vi "WPI_DMAEnableGlobal.vi"(9 "Set":bool, 10 "DMA Enable":T1) -> (1 "WordsPerSample":u16, 2 "DMA Enable Out":T1)   [LabVIEW 2017]
uses:
  <vilib>/Rock Robotics/SystemInterfaces/DMA/FPGA_DMAEnable.ctl
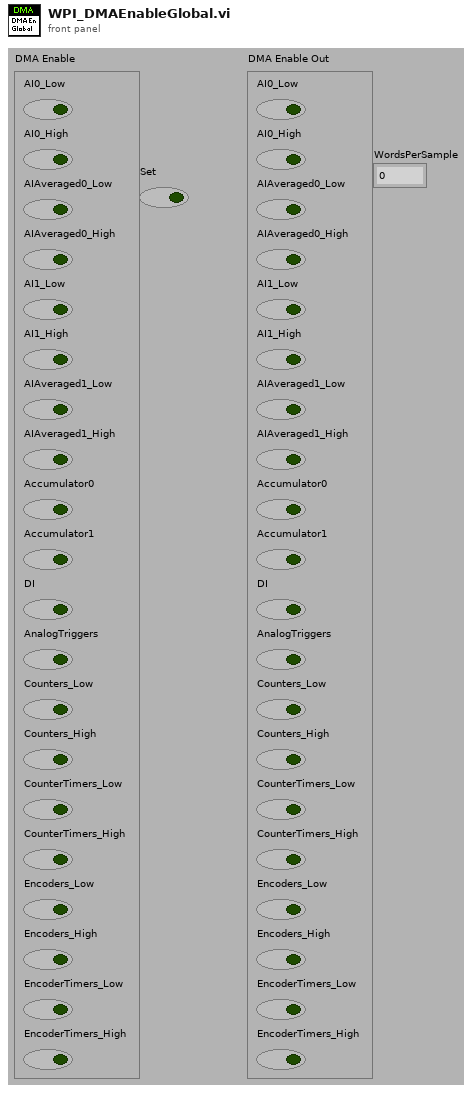
[diagram p1: front panel]
types:
  T1 = typedef "FPGA_DMAEnable.ctl" = cluster{"AI0_Low":bool, "AI0_High":bool, "AIAveraged0_Low":bool, "AIAveraged0_High":bool, "AI1_Low":bool, "AI1_High":bool, "AIAveraged1_Low":bool, "AIAveraged1_High":bool, "Accumulator0":bool, "Accumulator1":bool, "DI":bool, "AnalogTriggers":bool, "Counters_Low":bool, "Counters_High":bool, "CounterTimers_Low":bool, "CounterTimers_High":bool, "Encoders_Low":bool, "Encoders_High":bool, "EncoderTimers_Low":bool, "EncoderTimers_High":bool}
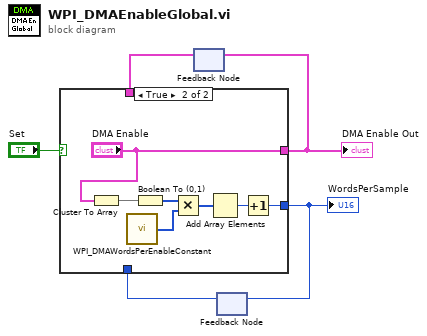
[diagram p0: block diagram]
diagram:
  n1 = feedback #1() -> (w3:T1)  [unwired: 1 out]
  n2 = feedback #2() -> (w1:i32)  [unwired: 1 out]
  n3 = case shown="True" "Set" {
    tunnel: [w7 "DMA Enable"] -> w4
    tunnel: w3 -> [w7 _]
    tunnel: [w6 w8] -> w2
    tunnel: w1 -> [w6 _]
    frame False {
    }
    frame True {
      n4 = Cluster To Array(cluster="DMA Enable") -> (array=w10:bool[])
      n5 = call <vilib>:"WPI_DMAWordsPerEnableConstant.vi"() -> ("WordsPerEnable"=w12:i32[])
      n6 = Boolean To (0,1)(Boolean=w10) -> (0, 1=w11:i16[])
      n7 = Multiply(x=w11, y=w12) -> (x*y=w13:i32[])
      n8 = Add Array Elements(numeric array=w13) -> (sum=w14:i32)
      n9 = Increment(x=w14) -> (x+1=w8:i32)
    }
  }
  "DMA Enable Out" <- w4
  "WordsPerSample" <- w2
  n10 = feedback-in #1(w4) -> ()
  n11 = feedback-in #2(w2) -> ()
